vi "Serpentine to Raster Image Conversion.vi"(10 "Input":i16[][](array[numeric])) -> (2 "Output":i16[][](array[numeric]))   [LabVIEW 2018]
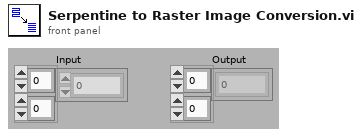
[diagram p1: front panel]
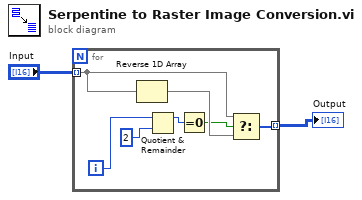
[diagram p0: block diagram]
diagram:
  n1 = for {
    tunnel: "Input" -> [w5] mode=indexing
    tunnel: [w6] -> w1 mode=indexing
    i -> [w9]
    n2 = Reverse 1D Array(array=w5) -> (reversed array=w4:i16[])
    n3 = Quotient & Remainder(x=w9, y=2) -> (x-y*floor(x/y)=w7:i32)  [unwired: 1 out]
    n4 = Equal To 0?(x=w7) -> (x = 0?=w3:bool)
    n5 = Select(t=w5, s=w3, f=w4) -> (s? t:f=w6:i16[])
  }
  "Output" <- w1
